vi "save.vi"(0 "VISA资源名称":refnum<visa-resource-name>, 5 "字符串":string) -> (4 "本次":string)   [LabVIEW 2017]
uses:
  <vilib>/Instr/_visa.llb/VISA Configure Serial Port (Instr).vi
  <vilib>/addons/Tools/Unicode/UTF8 Tools.lvlib
panel:
  out "错误输出 2":errorcluster caption="错误输出"
  in  "?":enum32{"CONTROL", "选项卡 2"}(tab)
  in  "增益选择":u16(ring) items=["±6.144V", "±4.096V", "±2.048V", "±1.024V", "±0.512V", "±0.256V"]
  in  "连接方式":u16(ring) items=["Serial", "WiFi", "Dual"]
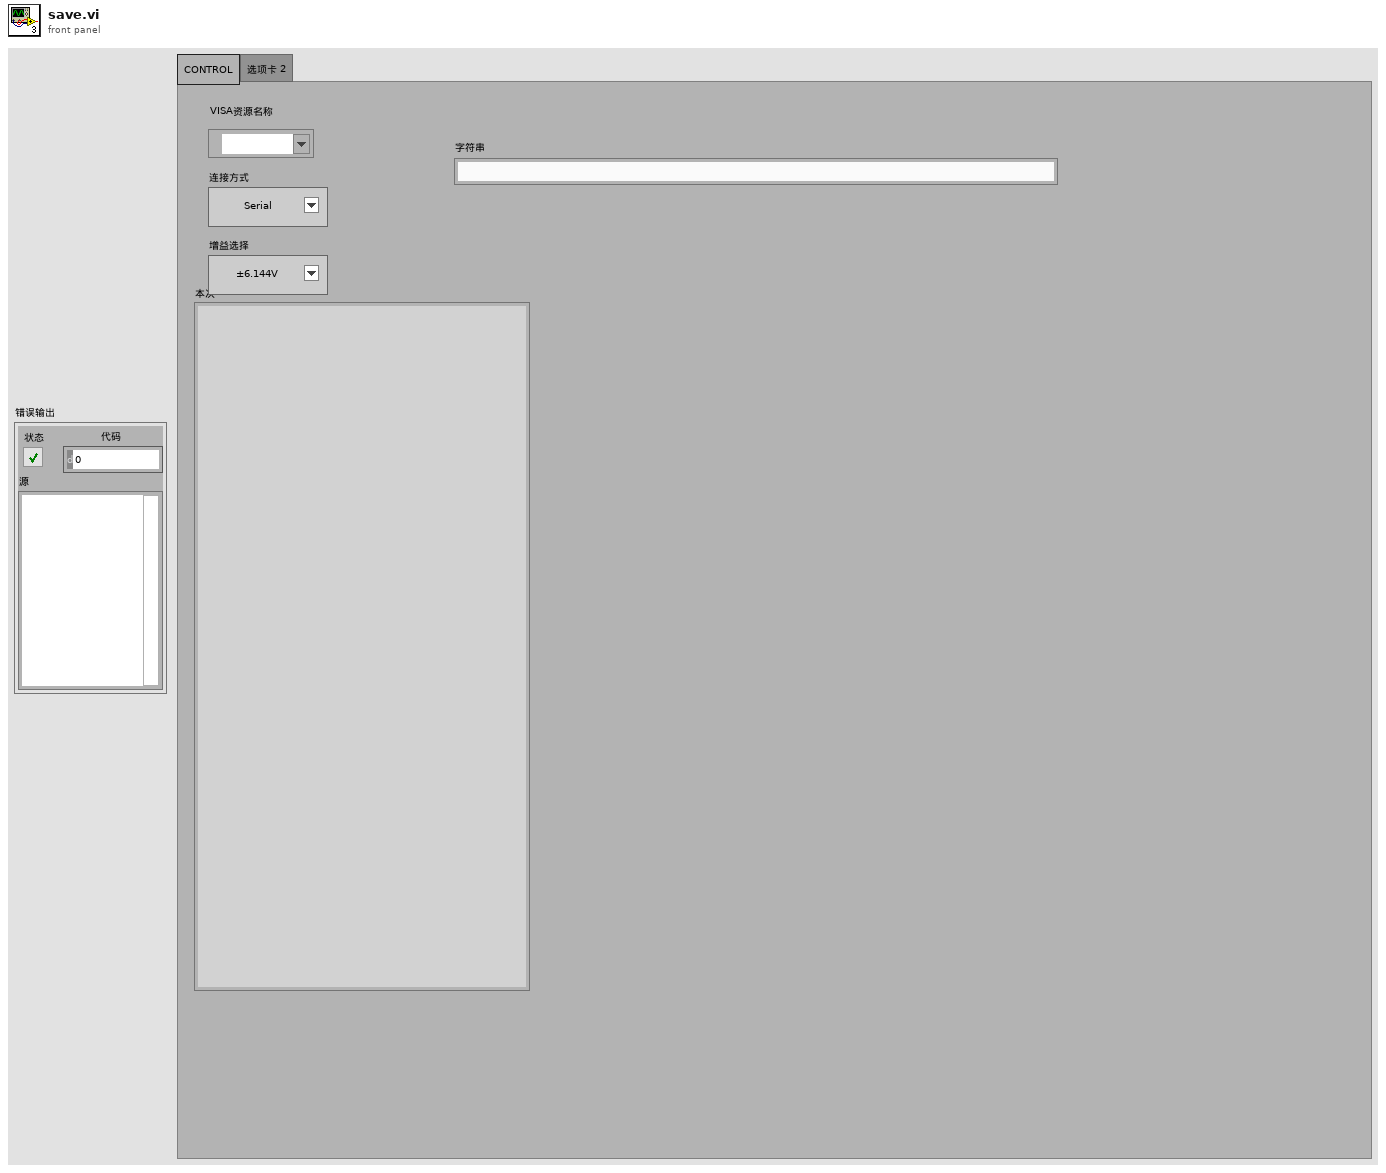
[diagram p1: front panel]
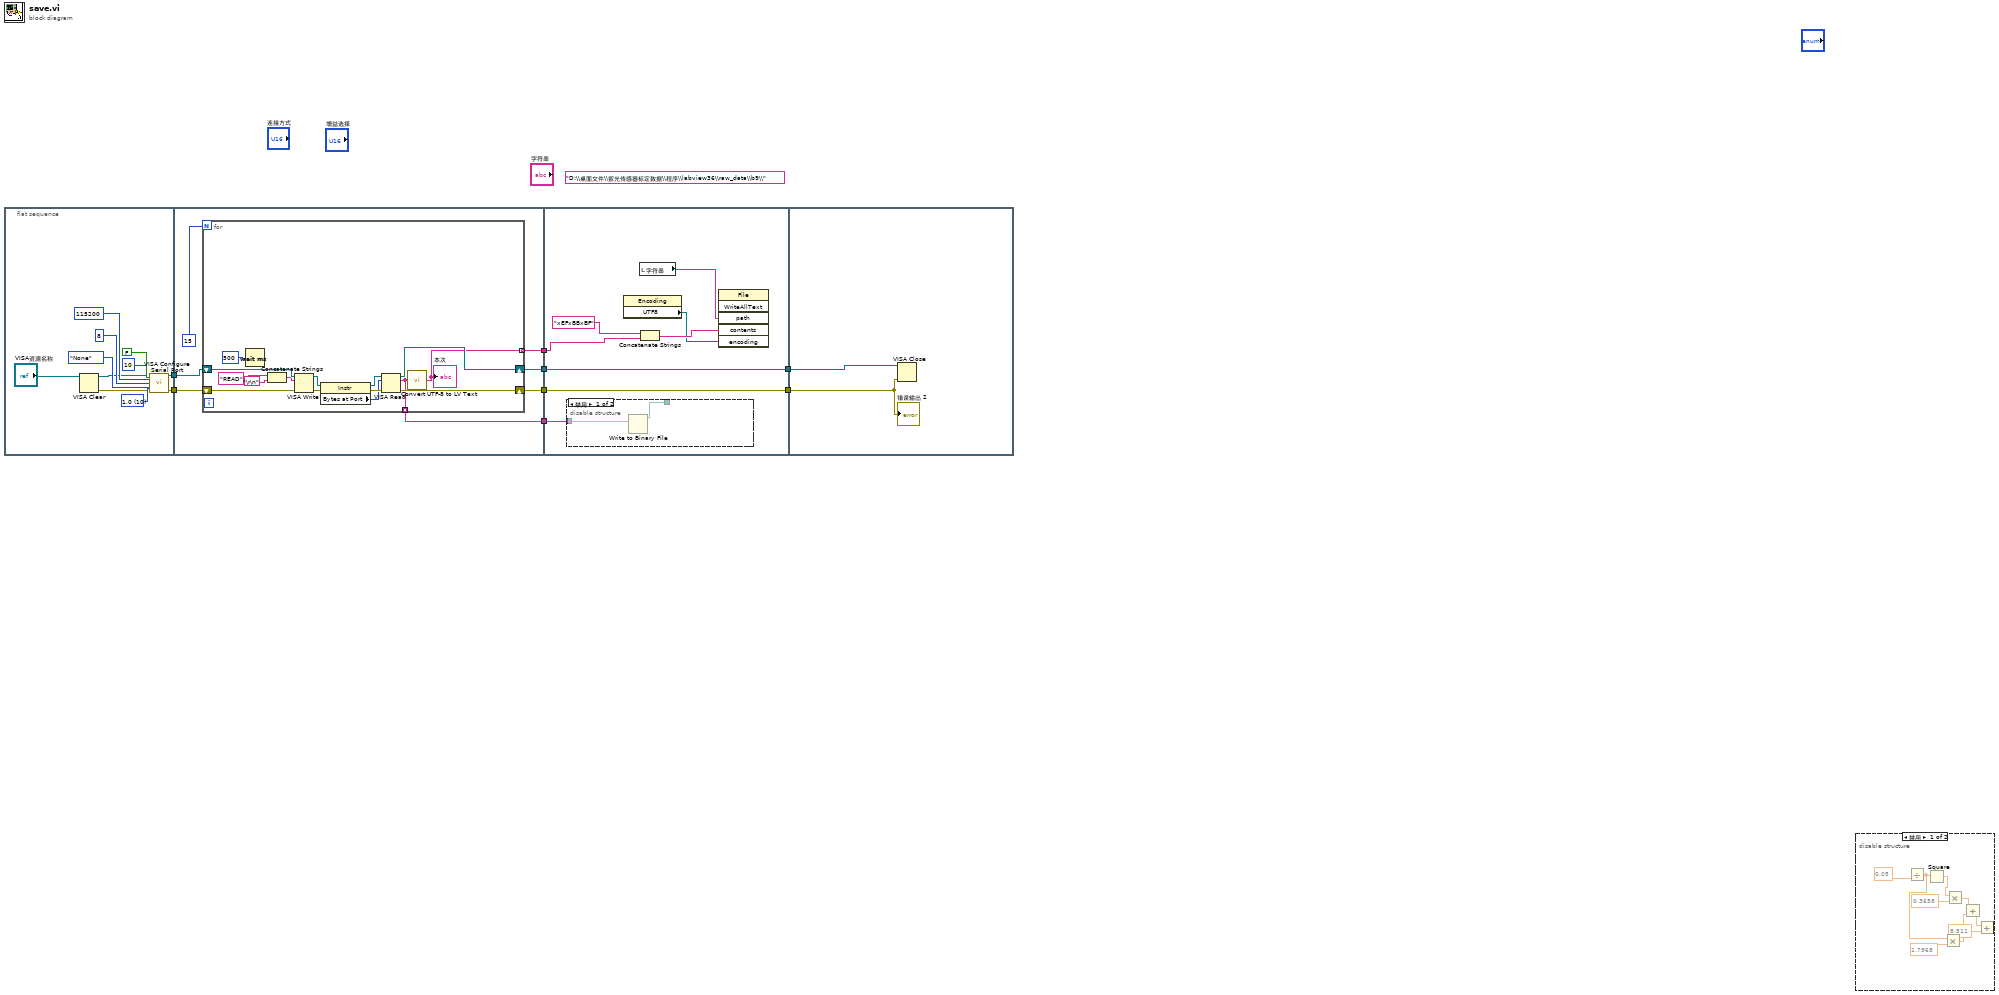
[diagram p0: block diagram]
diagram:
  (unwired) "D:\\桌面文件\\紫光传感器标定数据\\程序\\labview36\\raw_data\\b9\\"
  n1 = flat-sequence {
    tunnel: [w11] -> w8
    tunnel: [w10] -> w7
    tunnel: w8 -> [w26]
    tunnel: w7 -> [w25]
    tunnel: [w24] -> w6
    tunnel: [w23] -> w4
    tunnel: [w21] -> w2
    tunnel: [w20] -> w1
    tunnel: w6 -> [w49]
    tunnel: [w49] -> w5
    tunnel: w4 -> [w48]
    tunnel: [w48] -> w3
    tunnel: w2 -> [w47]
    tunnel: w1 -> [w46]
    tunnel: w5 -> [w53]
    tunnel: w3 -> [w52]
    frame #0 {
      w18 = u16 10 items=["1.0"=10, "1.5"=15, "2.0"=20] ("stop bits (10: 1 bit)")
      n2 = VISA Clear(VISA resource name="VISA资源名称") -> (VISA resource name out=w14:refnum<visa-resource-name>, error out=w13:errorcluster)  [unwired: 1 in]
      n3 = call-poly "VISA Configure Serial Port"("VISA resource name"=w14, "termination char\n(0xA = '\\n' = LF)"=u8 10 ("termination char\n(0xA = '\\n' = LF)"), "Enable Termination\nChar (T)"=FALSE ("Enable Termination\nChar (T)"), "baud rate (9600)"=u32 115200, "data bits (8)"=u16 8, "parity (0:none)"=enum16{"None", "Odd", "Even", "Mark", "Space"}."None", "error in (no error)"=w13, "stop bits (10: 1 bit)"=w18) -> ("VISA resource name out"=w10:refnum<visa-resource-name>, "error out"=w11:errorcluster)  [unwired: 6 in]
    }
    frame #1 {
      n4 = for {
        N: 15 -> [_]
        shift-right: [w38] -> w23
        shift-left: w26 -> [w41]
        shift-right: [w39] -> w24
        shift-left: w25 -> [w40]
        tunnel: [w28] -> w21 mode=indexing
        tunnel: [w27] -> w20 mode=indexing
        n5 = Wait (ms)(milliseconds to wait=u32 500 ("等待时间（毫秒）")) -> ()  [unwired: 1 out]
        n6 = Concatenate Strings("READ" ("字符串"), "\r\n") -> (w37:string)
        n7 = VISA Write(VISA resource name=w40, write buffer=w37, error in (no error)=w41) -> (VISA resource name out=w36:refnum<visa-resource-name>, error out=w35:errorcluster)  [unwired: 1 out]
        n8 = property class="Instr"(reference=w36, error in=w35) -> (reference out=w33:refnum<visa-resource-name>, error out=w32:errorcluster, "Bytes at Port"=w31:u32)
        n9 = VISA Read(VISA resource name=w33, byte count=w31, error in (no error)=w32) -> (VISA resource name out=w39:refnum<visa-resource-name>, read buffer=w27:string, error out=w38:errorcluster)  [unwired: 1 out]
        n10 = call <vilib>:"Convert UTF-8 to LV Text.vi"("UTF-8 Text"=w27) -> ("LV Text"=w28:string)  [unwired: 13 in, 1 out]
        "本次" <- w28
      }
    }
    frame #2 {
      n11 = disable-structure shown="禁用" {
        disable-tunnel: w46 -> [w51 _]
        disable-tunnel: _ -> [w50 _]
        frame Disabled {
          n12 = Write to Binary File(file (use dialog)=w50, data=w51) -> ()  [unwired: 4 in, 3 out]
        }
        frame Enabled {
        }
      }
      n13 = property class="Encoding"() -> ("UTF8"=w42:refnum<k24>)  [unwired: 2 in, 2 out]
      n14 = local read "字符串"() -> (w43:string)
      n15 = Concatenate Strings("xEFxBBxBF", w47) -> (w44:string)
      n16 = invoke on="调用节点" class="File" method="WriteAllText"("path"=w43, "contents"=w44, "encoding"=w42) -> ()  [unwired: 3 in, 6 out]
    }
    frame #3 {
      n17 = VISA Close(VISA resource name=w53, error in (no error)=w52) -> ()  [unwired: 1 out]
      "错误输出 2" <- w52
    }
  }
  n18 = disable-structure shown="禁用" {
    frame Disabled {
      n19 = Divide(y=0.05) -> (x/y=w58:dbl)  [unwired: 1 in]
      n20 = Square(x=w58) -> (x^2=w61:dbl)
      n21 = Multiply(x=w58, y=1.7968) -> (x*y=w56:dbl)
      n22 = Multiply(x=w61, y=0.3658) -> (x*y=w59:dbl)
      n23 = Add(x=w59, y=w56) -> (x+y=w55:dbl)
      n24 = Add(x=w55, y=8.511) -> ()  [unwired: 1 out]
    }
    frame Enabled {
    }
  }
